vi "Determine Next State.vi"(4 "Status?":bool, 7 "Previous State":string) -> (0 "New State":string, 3 "Remaining States":string)   [LabVIEW 2011]
panel:
  # "[Title] - [DESCRIPTION]\n\nCopyright (C) 2004 Michael Aivaliotis michael@mmwis.com\n\nPlease visit http://www.OpenG.org to learn about the\nOpen Source LabVIEW software movement.\n\nThis library is free software; you can redistribute it and/or\nmodify it under the terms of the GNU Lesser General Public\nLicense as published by the Free Software Foundation; either\nversion 2.1 of the License, or (at your option) any later version.\nThis library is distributed in the hope that it will be useful,\nbut WITHOUT ANY WARRANTY; without even the implied warranty of\nMERCHANTABILITY or FITNESS FOR A PARTICULAR PURPOSE. See the GNU\nLesser General Public License for more details.\nYou should have received a copy of the GNU Lesser General Public\nLicense along with this library; if not, write to the Free Software\nFoundation, Inc., 59 Temple Place, Suite 330, Boston, MA 02111-1307 USA"
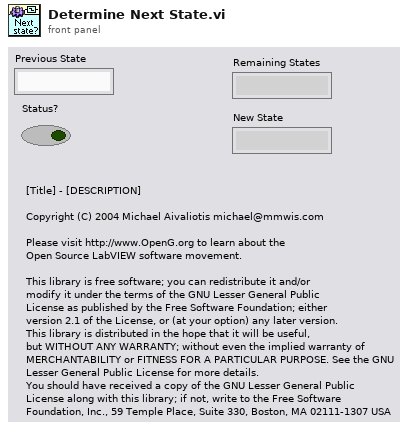
[diagram p1: front panel]
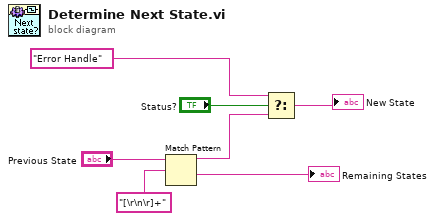
[diagram p0: block diagram]
diagram:
  n1 = Match Pattern(string="Previous State", regular expression="[\r\n\r]+" ("Substring")) -> (before substring=w5:string, after substring=→"Remaining States":string)  [unwired: 3 out]
  n2 = Select(t="Error Handle", s="Status?", f=w5) -> (s? t:f=→"New State":string)
